vi "DDS Read Register.vi"(6 "channel number (1)":u8=1 min=1 max=4 step=1, 8 "error in (no error)":errorcluster, 10 "Register":T3, 11 "DDS ref in":T1={"NI USB-8451 device reference"="", "DIO port"=0, "Serial Clock Rate [kHz]"=1000}) -> (0 "error out":errorcluster, 2 "Read data":u8[](array[numeric]), 3 "DDS ref out":T1={"NI USB-8451 device reference"="", "DIO port"=0, "Serial Clock Rate [kHz]"=1000})   [LabVIEW 2013]
doc: "Reads the current value of the specified register in the specified channel. Note that only the profile register currently selected by the external profile pins can be read."
uses:
  AD9910 registers.ctl
  DDS_box_device_reference.ctl
  <vilib>/ni845x/ni845x.llb/ni845xControl.ctl
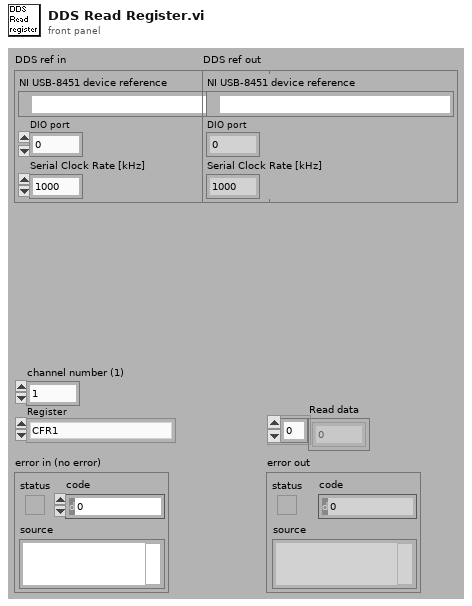
[diagram p1: front panel]
types:
  T1 = typedef "DDS_box_device_reference.ctl" = cluster{"NI USB-8451 device reference":T2, "DIO port":u8, "Serial Clock Rate [kHz]":u16}
  T2 = typedef "ni845xControl.ctl" = refnum<k21>
  T3 = typedef "AD9910 registers.ctl" = enum16{"CFR1", "CFR2", "CFR3", "Auxiliary DAC Control", "I/0 Update Rate", "Frequency Tuning Word", "Phase Offset Word", "Amplitude Scale Factor", "Multichip Sync", "Digital Ramp Limit", "Digital Ramp Step Size", "Digital Ramp Rate", "Single Tone Profile 0", "Single Tone Profile 1", "Single Tone Profile 2", "Single Tone Profile 3", "Single Tone Profile 4", "Single Tone Profile 5", "Single Tone Profile 6", "Single Tone Profile 7", "RAM Profile 0", "RAM Profile 1", "RAM Profile 2", "RAM Profile 3", "RAM Profile 4", "RAM Profile 5", "RAM Profile 6", "RAM Profile 7", "RAM"}
  T4 = typedef "ni845xSpiScriptControl.ctl" = refnum<k20>
  T5 = typedef "DDS CS pins.ctl" = enum8{"IO reset", "Ch. 4 CS", "Ch. 3 CS", "Ch. 2 CS", "Ch. 1 CS"}
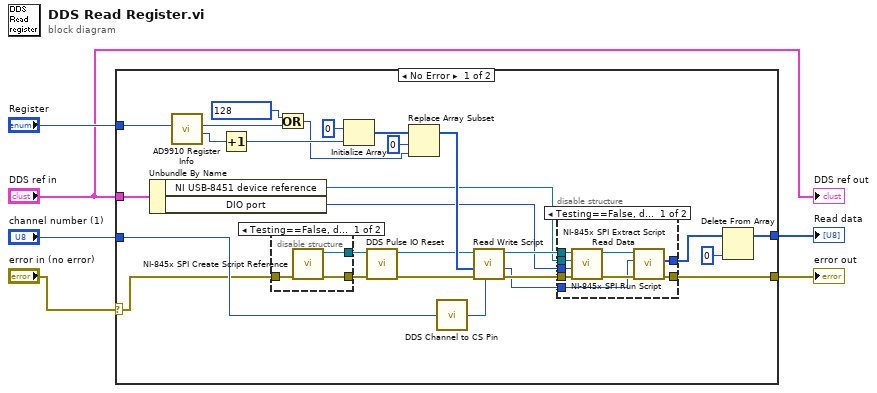
[diagram p0: block diagram]
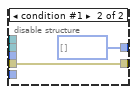
[diagram p2: hidden frame]
diagram:
  n1 = case shown="No Error" "error in (no error)" {
    selector: "error in (no error)" -> [w7 w49]
    tunnel: "DDS ref in" -> [w33 _]
    tunnel: "Register" -> [w30 _]
    tunnel: [w16 w49] -> w4
    tunnel: [w11 _] -> w3
    tunnel: "channel number (1)" -> [w9 _]
    frame No Error {
      n2 = Unbundle By Name(w33) -> ("NI USB-8451 device reference"=w19:T2, "DIO port"=w18:u8)
      n3 = call "AD9910 Register Info.vi"("Register"=w30) -> ("Number of Bytes"=w28:i32, "Address"=w15:u8)  [unwired: 9 in]
      n4 = Increment(x=w28) -> (x+1=w22:i32)
      n5 = disable-structure shown="Testing==False, default" {
        disable-tunnel: w7 -> [w47 w48]
        disable-tunnel: [w46 _] -> w32
        disable-tunnel: [w45 w48] -> w31
        frame condition #0 (active) {
          n6 = call <vilib>:"NI-845x SPI Create Script Reference.vi"("error in (no error)"=w47) -> ("error out"=w45:errorcluster, "spi script reference"=w46:T4)  [unwired: 9 in]
        }
        frame condition #1 {
        }
      }
      n7 = Or(x=u8 128, y=w15) -> (x .or. y?=w13:u8)
      n8 = Initialize Array(u8 0 ("element"), w22) -> (w27:u8[])
      n9 = call "DDS Pulse IO Reset.vi"("error in (no error)"=w31, "spi script reference in"=w32) -> ("error out"=w24:errorcluster, "spi script reference out"=w23:T4)  [unwired: 8 in]
      n10 = Replace Array Subset(array=w27, new element=w13, index=0) -> (w25:u8[])
      n11 = call "DDS Channel to CS Pin.vi"("channel number (1)"=w9) -> ("CS pin"=w8:T5)
      n12 = call "Read Write Script.vi"("chip select (0)"=w8, "error in (no error)"=w24, "Write Data"=w25, "spi script reference in"=w23) -> ("error out"=w21:errorcluster, "script read index"=w17:u32, "spi script reference out"=w20:T4)  [unwired: 5 in]
      n13 = disable-structure shown="Testing==False, default" {
        disable-tunnel: w21 -> [w42 w44]
        disable-tunnel: w20 -> [w41 _]
        disable-tunnel: w19 -> [w40 _]
        disable-tunnel: w18 -> [w39 _]
        disable-tunnel: w17 -> [w36 _]
        disable-tunnel: [w35 w44] -> w16
        disable-tunnel: [w34 u8[] [] ("read data")] -> w12
        frame condition #0 (active) {
          n14 = call <vilib>:"NI-845x SPI Run Script.vi"("error in (no error)"=w42, "port (0)"=w39, "device reference in"=w40, "spi script reference in"=w41) -> ("error out"=w38:errorcluster, "spi script reference out"=w37:T4)  [unwired: 5 in, 1 out]
          n15 = call <vilib>:"NI-845x SPI Extract Script Read Data.vi"("error in (no error)"=w38, "script read index"=w36, "spi script reference in"=w37) -> ("error out"=w35:errorcluster, "read data"=w34:u8[])  [unwired: 6 in, 1 out]
        }
        frame condition #1 {
        }
      }
      n16 = Delete From Array(array=w12, index=0) -> (array with subset deleted=w11:u8[])  [unwired: 1 in, 1 out]
    }
    frame Error {
    }
  }
  "error out" <- w4
  "Read data" <- w3
  "DDS ref out" <- "DDS ref in"
